vi "Is Printable Character.vi"(1 "ASCII character":u8 format="%02x") -> (0 "True = the input is a Printable ASCII character (0x20 to 0x7F)":bool)   [LabVIEW 2020, in "Error Manager.lvlib"]
doc: "Returns True if and only if the input byte (ASCII character) represents a Printable Character.\n\nThere are 96 Printable Characters (ASCII hex values 0x20 to 0x7F)\n\nASCII table: https://www.ascii-code.com/\n\nPerformance: This VI is inlined to increase performance"
uses:
  Error Manager.lvlib
panel:
  # "Development\ncontrols/indicators useful for development and testing, but which are not outputs of the VI"
  # "Input\nInputs to the VI"
  # "Output\nOutputs of the VI"
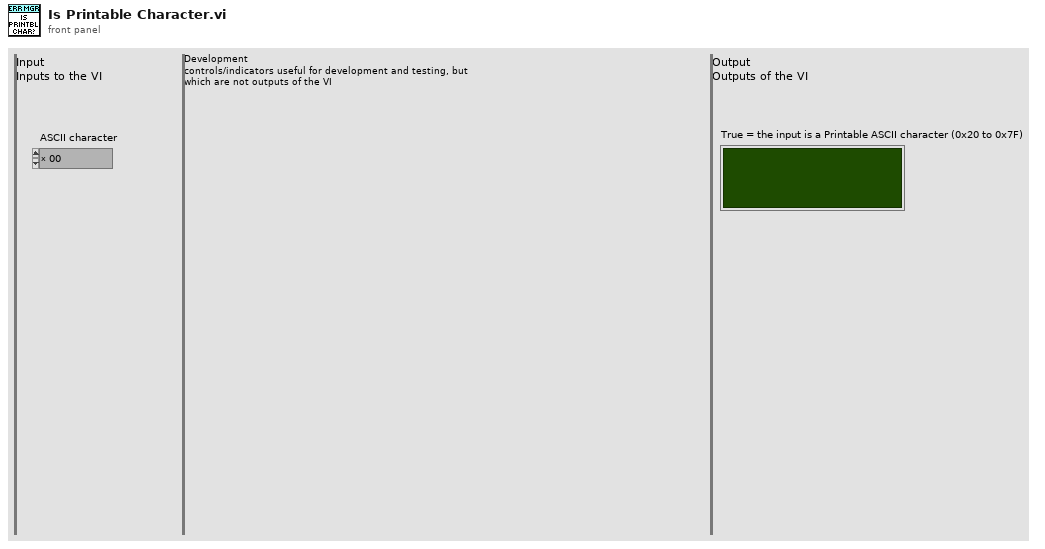
[diagram p1: front panel]
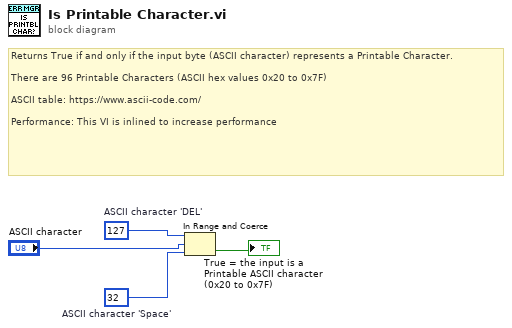
[diagram p0: block diagram]
diagram:
  w3 = u8 32  # ASCII character 'Space'
  w4 = u8 127  # ASCII character 'DEL'
  # "Returns True if and only if the input byte (ASCII character) represents a Printable Character.\n\nThere are 96 Printable Characters (ASCII hex values 0x20 to 0x7F)\n\nASCII table: https://www.ascii-code.com/\n\nPerformance: This VI is inlined to increase performance"
  n1 = In Range and Coerce(upper limit=w4, x="ASCII character", lower limit=w3) -> (In Range?=→"True = the input is a Printable ASCII character (0x20 to 0x7F)":bool)  [unwired: 1 out]
